vi "test.write_log.vi"   [LabVIEW 2020]
uses:
  Nominal Client/Nominal Client.lvclass/Nominal Client.ctl
  <vilib>/numeric/Random Number (Range) I64.vi
  990e7071-dbe3-43dc-84d2-0d074c4f9026.vi
  <vilib>/numeric/sub_Random U32.vi
  Nominal Client/private_data.set.vi
  990e7071-dbe3-43dc-84d2-0d074c4f9026.vi/8284acbc-2d4d-4b18-b492-8ff51a6e7e10.vi
  nominal types/workspace/id.get.vi
  nominal types/workspace/rid.get.vi
  <vilib>/AdvancedString/1D String Array to Delimited String.vi
  Nominal Client/workspace.set.vi
  <vilib>/Utility/file.llb/Application Directory.vi
  <vilib>/Utility/error.llb/Error Cluster From Error Code.vi
  Nominal Client/format endpoint termination.vi
  submodules/reqwest-labview/lv-src/reqwest/create.vi
  Nominal Client/workspace_cache.get_from_rid.vi
  Nominal Client/workspace_cache.get.vi
  Nominal Client/Palette Items/who_am_i.vi
  User/User.lvclass
  Nominal Client/Nominal Client.lvclass
  nominal types/workspace/workspace.lvclass
  submodules/reqwest-labview/lv-src/reqwest/reqwest.lvclass
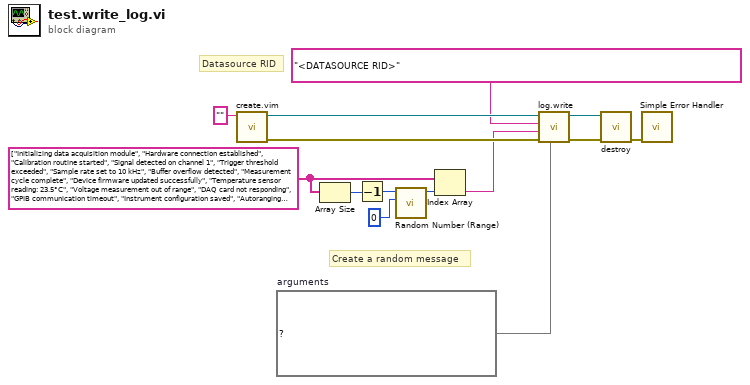
[diagram p0: block diagram]
diagram:
  w1 = map{string, string} {"channel"="24.0", "configuration"="Test Stand A", "current"="Baseline", "cycle_count"="Modified", "equipment_id"="100.3", "firmware_version"="1000", "flow_rate"="Config 1", "location"="120", "mode"="240", "operator"="John Smith", "pressure_setpoint"="Test Stand C", "run_number"="12.5", "severity"="v2.0.1", "software_version"="500", "status"="v1.2.3", "subsystem"="fw_3.4.0", "temperature_setpoint"="Test Stand B", "test_id"="25.5", "test_stand"="Jane Doe", "voltage"="Config 2"}  # arguments
  w4 = string[] ["Initializing data acquisition module", "Hardware connection established", "Calibration routine started", "Signal detected on channel 1", "Trigger threshold exceeded", "Sample rate set to 10 kHz", "Buffer overflow detected", "Measurement cycle complete", "Device firmware updated successfully", "Temperature sensor reading: 23.5°C", "Voltage measurement out of range", "DAQ card not responding", "GPIB communication timeout", "Instrument configuration saved", "Autoranging enabled for channel 2", "Waveform capture initiated", "Data logging started", "Hardware self-test passed", "Analog input configuration applied", "Digital output state changed", "Synchronization pulse detected", "Acquisition stopped by user", "Channel 3 disabled", "Offset compensation applied", "Gain adjusted for optimal range", "External trigger configured", "Memory buffer cleared", "Sampling clock configured", "Hardware error: Check connections", "Reference voltage stable", "Shunt resistor value updated", "Input impedance set to 1 MO", "Filter settings applied", "Averaging mode enabled", "Peak detection threshold set", "Instrument warming up", "Measurement accuracy within spec", "Data transfer to host complete", "Channel coupling set to DC", "Hardware interrupt received", "Probe compensation required", "Signal conditioning applied", "Noise floor measurement complete", "Oversampling ratio set to 16x", "Hardware timer configured", "Burst mode enabled", "Continuous acquisition started", "Module temperature normal", "Input protection activated", "Calibration certificate expires soon", "Bandwidth limit applied", "Measurement uncertainty calculated", "Hardware watchdog reset", "Signal integrity verified", "Pretrigger buffer configured", "Analog filter bypassed", "Hardware synchronization established", "Data decimation applied", "Channel crosstalk within limits", "Instrument identity verified", "Trigger mode set to edge", "Sample clock jitter measured", "Hardware FIFO nearly full", "Measurement statistics updated", "Auto-zero correction applied", "Input range changed to ±10V", "Hardware capabilities queried", "Waveform analysis complete", "Channel enabled for acquisition", "Power supply voltage nominal", "External clock reference locked", "Data streaming active", "Hardware revision detected", "Measurement interval set", "Trigger holdoff configured", "Signal amplitude measured", "Hardware reset performed", "Input bias current compensated", "Acquisition rate limited by hardware", "Channel label updated", "Measurement units set to Volts", "Hardware buffer allocated", "Timestamp synchronization enabled", "Trigger position adjusted", "Signal-to-noise ratio calculated", "Module slot identification complete", "Hardware interlock engaged", "Data compression enabled", "Channel sensitivity adjusted", "Measurement range verification failed", "Input signal clipped", "Hardware diagnostics running", "Probe attenuation factor applied", "Acquisition memory optimized", "Trigger source selected", "Signal frequency detected", "Hardware cooling fan operational", "Measurement alarm threshold set"] ("string array")
  # "Create a random message"
  # "Datasource RID"
  n1 = call "create.vim"("API Token (string or path)"="") -> ("error out"=w11:errorcluster, "Nominal Client"=w12:refnum<class "Nominal Client.lvclass">)  [unwired: 8 in, 1 out]
  n2 = Array Size(array=w4) -> (size(s)=w7:i32)
  n3 = Decrement(x=w7) -> (x-1=w6:i32)
  n4 = call-poly <vilib>:"Random Number (Range).vi"("lower bound (-100)"=i64 0, "upper bound (100)"=w6) -> ("number"=w5:i64)  [unwired: 9 in]
  n5 = Index Array(array=w4, index=w5) -> (element=w3:string)
  n6 = call "log.write.vi"("Arguments"=w1, "error in"=w11, "Message"=w3, "dataSourceRid"="<DATASOURCE RID>" ("Asse"), "Nominal Client in"=w12) -> ("error out"=w9:errorcluster, "Nominal Client out"=w10:refnum<class "Nominal Client.lvclass">)  [unwired: 5 in]
  n7 = call "destroy.vi"("error in"=w9, "Nominal Client"=w10) -> ("error out"=w13:errorcluster)  [unwired: 9 in]
  n8 = call <vilib>:"Simple Error Handler.vi"("error in (no error)"=w13) -> ()  [unwired: 4 in, 5 out]
